vi "make_lut_lookup.vi"(9 "Calibration data":T1, 11 "LUT inputs":sgl[](array[numeric])) -> (1 "In range":bool, 3 "XYZ and match error":sgl[](array[numeric]))   [LabVIEW 2012]
uses:
  initialization/asap_calibration.ctl
  <vilib>/Analysis/Matrix/Datatypes/RealMatrix.ctl
  <vilib>/Analysis/Matrix/NI_Matrix.lvlib
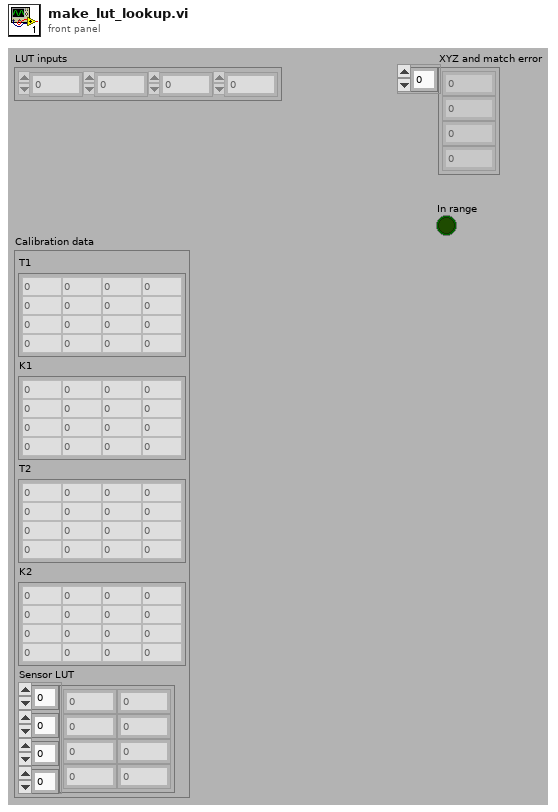
[diagram p1: front panel]
types:
  T1 = typedef "asap_calibration.ctl" = cluster{"T1":T2, "K1":T2, "T2":T2, "K2":T2, "Sensor LUT":sgl[][][][]}
  T2 = typedef "NI_Matrix.lvlib/RealMatrix.ctl" = dbl[][]
  T3 = cluster{"X values":waveform(dbl), "Y values":waveform(dbl), "Z values":waveform(dbl)}
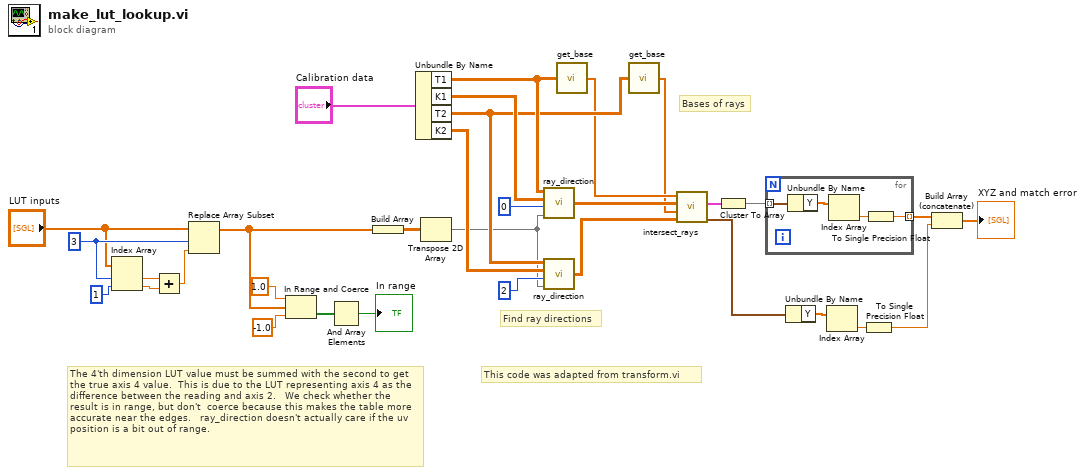
[diagram p0: block diagram]
diagram:
  w13 = 3 ("index (row)")
  # "This code was adapted from transform.vi"
  # "The 4'th dimension LUT value must be summed with the second to get the true axis 4 value.  This is due to the LUT representing axis 4 as the difference between the reading and axis 2.   We check whether the result is in range, but don't  coerce because this makes the table more accurate near the edges.   ray_direction doesn't actually care if the uv position is a bit out of range."
  # "Bases of rays"
  # "Find ray directions"
  n1 = Index Array(array="LUT inputs", index #1=w13, index #2=1 ("index (row)")) -> (element #1=w11:sgl, element #2=w10:sgl)
  n2 = Add(x=w11, y=w10) -> (x+y=w9:sgl)
  n3 = Replace Array Subset(array="LUT inputs", new element=w9, index=w13) -> (w1:sgl[])
  n4 = In Range and Coerce(upper limit=sgl 1.0, x=w1, lower limit=sgl -1.0) -> (In Range?=w7:bool[])  [unwired: 1 out]
  n5 = And Array Elements(Boolean array=w7) -> (logical AND=→"In range":bool)
  n6 = Build Array(w1) -> (w5:sgl[][])
  n7 = Unbundle By Name("Calibration data") -> ("T1"=w25:T2, "K1"=w24:T2, "T2"=w23:T2, "K2"=w22:T2)
  n8 = Transpose 2D Array(2D array=w5) -> (transposed array=w4:sgl[][])
  n9 = call "ray_direction.vi"("Axis positions"=w4, "first axis"=0 ("index"), "K"=w24, "T"=w25) -> ("Ray directions"=w27:T2)  [unwired: 2 out]
  n10 = call "ray_direction.vi"("Axis positions"=w4, "first axis"=2 ("index"), "K"=w22, "T"=w23) -> ("Ray directions"=w26:T2)  [unwired: 2 out]
  n11 = call "get_base.vi"("T"=w25) -> ("Array"=w21:dbl[])
  n12 = call "get_base.vi"("T"=w23) -> ("Array"=w20:dbl[])
  n13 = call "intersect_rays.vi"("Sensor 2 directions"=w26, "Sensor 2 base"=w20, "Sensor 1 directions"=w27, "Sensor 1 base"=w21) -> ("Match error"=w17:waveform(dbl), "XYZ"=w31:T3)  [unwired: 2 in, 4 out]
  n14 = Cluster To Array(cluster=w31) -> (array=w32:waveform(dbl)[])
  n15 = for {
    tunnel: w32 -> [w36] mode=indexing
    tunnel: [w33] -> w16 mode=indexing
    n16 = Unbundle By Name(w36) -> ("Y"=w35:dbl[])
    n17 = Index Array(array=w35) -> (element=w34:dbl)  [unwired: 1 in]
    n18 = To Single Precision Float(number=w34) -> (single precision float=w33:sgl)
  }
  n19 = Unbundle By Name(w17) -> ("Y"=w18:dbl[])
  n20 = Index Array(array=w18) -> (element=w19:dbl)  [unwired: 1 in]
  n21 = To Single Precision Float(number=w19) -> (single precision float=w14:sgl)
  n22 = Build Array (concatenate)(w16, w14) -> (→"XYZ and match error":sgl[])
